vi "dfd_Group Delay_Params Validation.vi"(4 "max pole radius (in)":dbl=0.95 min=0.0, 6 "fs [Hz]":dbl=1.0 format="%.2f", 7 "parameters":T1={"iteration"={"epsilon"=1e-05, "times"=300}, "initial guess"={"iteration times"=5, "seed"=1.0}}, 8 "error in (no error)":errorcluster, 9 "p (in)":i32=128, 10 "dfd_Group Delay_Band Spec":T2[](array[typedef]) {"subband specs"."weight" format="%.2f"}, 11 "order":i32) -> (0 "error out":errorcluster, 1 "p (out)":i32=128, 2 "dfd_Group Delay_Band Spec (dup)":T2[](array[typedef]) {"subband specs"."weight" format="%.2f"}, 3 "max pole radius (out)":dbl)   [LabVIEW 2017, in "NI_DigFilter_Design.lvlib"]
uses:
  <vilib>/addons/Digital Filter Design/NI_DigFilter_Design.lvlib
  <vilib>/addons/Digital Filter Design/_GroupDelay.llb/dfd_Group Delay_Band Spec.ctl
  <vilib>/addons/Digital Filter Design/_Misc.llb/dfd_Error Handlers (Multiple).vi
  <vilib>/addons/Digital Filter Design/NI_DigFilterLicensed.lvlib
panel:
  # "freq"
  # "group delay"
  # "weight"
  # "freq"
  # "group delay"
  # "weight"
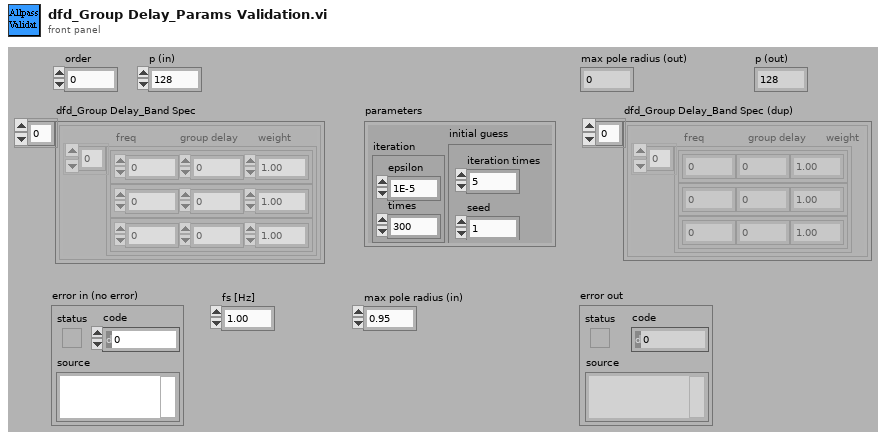
[diagram p1: front panel]
types:
  T1 = cluster{"iteration":cluster{"epsilon":dbl, "times":i32}, "initial guess":cluster{"iteration times":i32, "seed":dbl}}
  T2 = typedef "NI_DigFilterLicensed.lvlib/dfd_Group Delay_Band Spec.ctl" = cluster{"subband specs":cluster{"freq":dbl, "group delay":dbl, "weight":dbl}[]}
  T3 = cluster{"freq":dbl, "group delay":dbl, "weight":dbl}[]
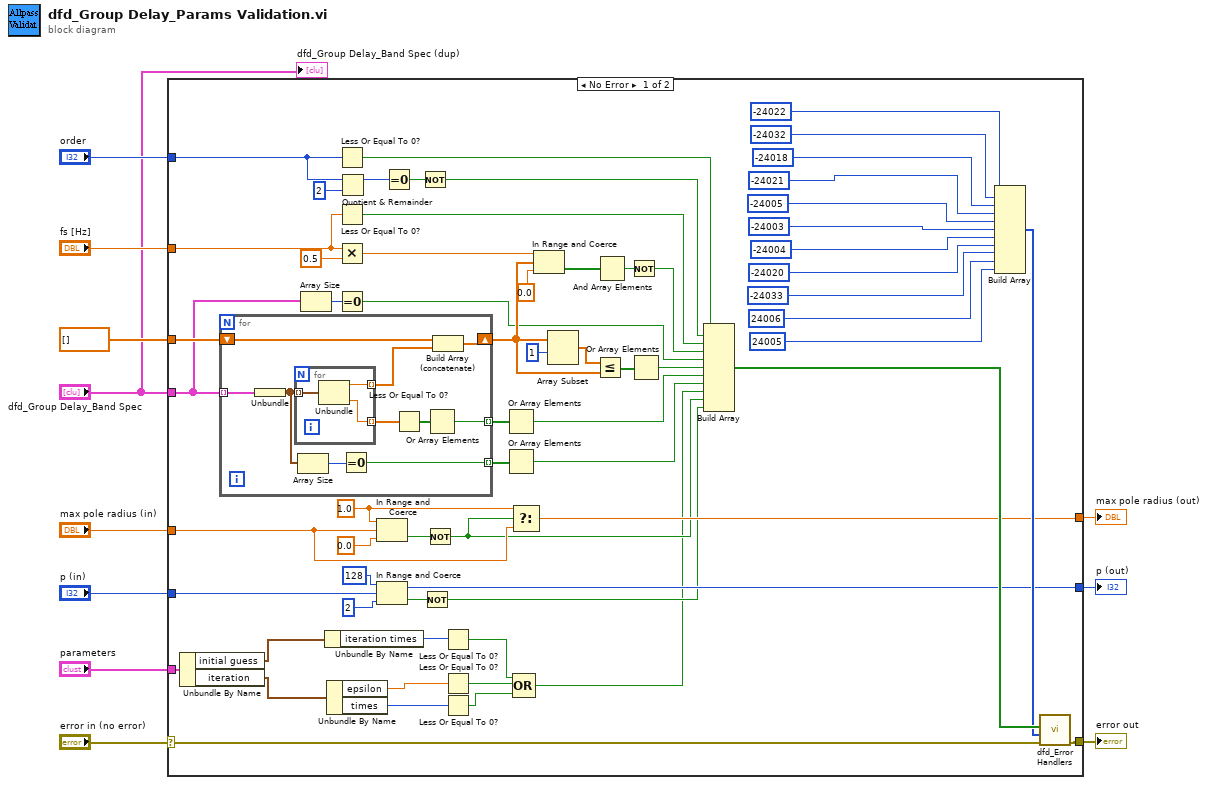
[diagram p0: block diagram]
diagram:
  n1 = case shown="No Error" "error in (no error)" {
    selector: "error in (no error)" -> [w54 w90]
    tunnel: dbl[] [] -> [w75 _]
    tunnel: "fs [Hz]" -> [w62 _]
    tunnel: [w59 w90] -> w9
    tunnel: "p (in)" -> [w44 w91]
    tunnel: [w43 w91] -> w7
    tunnel: "dfd_Group Delay_Band Spec" -> [w42 _]
    tunnel: "order" -> [w28 _]
    tunnel: "max pole radius (in)" -> [w36 w89]
    tunnel: [w34 w89] -> w2
    tunnel: "parameters" -> [w18 _]
    frame No Error {
      w35 = 1.0 ("upper limit")
      n2 = Unbundle By Name(w18) -> ("initial guess"=w20:cluster{"iteration times":i32, "seed":dbl}, "iteration"=w19:cluster{"epsilon":dbl, "times":i32})
      n3 = for {
        tunnel: w42 -> [w85] mode=indexing
        shift-right: [w82] -> w68
        shift-left: w75 -> [w84]
        tunnel: [w79] -> w71 mode=indexing
        tunnel: [w76] -> w48 mode=indexing
        n4 = Unbundle(w85) -> ("subband specs"=w78:T3)
        n5 = for {
          tunnel: w78 -> [w88] mode=indexing
          tunnel: [w87] -> w83 mode=indexing
          tunnel: [w86] -> w81 mode=indexing
          n6 = Unbundle(w88) -> ("freq"=w87:dbl, "weight"=w86:dbl)  [unwired: 1 out]
        }
        n7 = Array Size(array=w78) -> (size(s)=w77:i32)
        n8 = Equal To 0?(x=w77) -> (x = 0?=w76:bool)
        n9 = Less Or Equal To 0?(x=w81) -> (x <= 0?=w80:bool[])
        n10 = Or Array Elements(Boolean array=w80) -> (logical OR=w79:bool)
        n11 = Build Array (concatenate)(w84, w83) -> (w82:dbl[])
      }
      n12 = Array Size(array=w42) -> (size(s)=w41:i32)
      n13 = Unbundle By Name(w20) -> ("iteration times"=w37:i32)
      n14 = Unbundle By Name(w19) -> ("epsilon"=w33:dbl, "times"=w32:i32)
      n15 = Less Or Equal To 0?(x=w28) -> (x <= 0?=w25:bool)
      n16 = Less Or Equal To 0?(x=w62) -> (x <= 0?=w60:bool)
      n17 = Multiply(x=w62, y=0.5) -> (x*y=w64:dbl)
      n18 = Equal To 0?(x=w41) -> (x = 0?=w39:bool)
      n19 = Quotient & Remainder(x=w28, y=2) -> (x-y*floor(x/y)=w26:i32)  [unwired: 1 out]
      n20 = In Range and Coerce(upper limit=w35, x=w36, lower limit=0.0) -> (In Range?=w45:bool)  [unwired: 1 out]
      n21 = In Range and Coerce(upper limit=128, x=w44, lower limit=2) -> (coerced(x)=w43:i32, In Range?=w56:bool)
      n22 = Equal To 0?(x=w26) -> (x = 0?=w24:bool)
      n23 = Not(x=w24) -> (.not. x?=w21:bool)
      n24 = Not(x=w56) -> (.not. x?=w14:bool)
      n25 = Not(x=w45) -> (.not. x?=w13:bool)
      n26 = Less Or Equal To 0?(x=w37) -> (x <= 0?=w31:bool)
      n27 = Less Or Equal To 0?(x=w33) -> (x <= 0?=w30:bool)
      n28 = Less Or Equal To 0?(x=w32) -> (x <= 0?=w29:bool)
      n29 = Or Array Elements(Boolean array=w71) -> (logical OR=w66:bool)
      n30 = Or Array Elements(Boolean array=w48) -> (logical OR=w47:bool)
      n31 = Select(t=w35, s=w13, f=w36) -> (s? t:f=w34:dbl)
      n32 = Compound Arithmetic op=OR(w31, w30, w29) -> (w12:bool)
      n33 = In Range and Coerce(upper limit=w64, x=w68, lower limit=0.0) -> (In Range?=w73:bool[])  [unwired: 1 out]
      n34 = Array Subset(array=w68, index=1) -> (w69:dbl[])  [unwired: 1 in]
      n35 = Less Or Equal?(x=w69, y=w68) -> (x <= y?=w67:bool[])
      n36 = And Array Elements(Boolean array=w73) -> (logical AND=w72:bool)
      n37 = Not(x=w72) -> (.not. x?=w61:bool)
      n38 = Or Array Elements(Boolean array=w67) -> (logical OR=w40:bool)
      n39 = Build Array(w25, w21, w60, w61, w39, w40, w66, w47, w12, w13, w14) -> (w65:bool[])
      n40 = Build Array(-24022 ("ERR_ORDER_LE_ZERO"), -24032 ("ERR_ORDER_ODD"), -24018 ("ERR_FS_LE_ZERO"), -24021 ("ERR_FREQ_RANGE_WRONG"), -24005 ("ERR_EMPTY_BAND"), -24003 ("ERR_BAND_FREQ_SEG_WRONG"), -24004 ("ERR_WEIGHT_LE_ZERO"), -24020 ("ERR_INVALID_BAND"), -24033 ("ERR_INVALID_PARAMETERS"), 24006 ("WRN_RAIUS_RANGE"), 24005 ("WRN_P_RANGE")) -> (w49:i32[])
      n41 = call-poly <vilib>:"dfd_Error Handlers.vi"("error in (no error)"=w54, "error sources"=w49, "condition failed?"=w65) -> ("error out"=w59:errorcluster)  [unwired: 8 out]
    }
    frame Error {
    }
  }
  "error out" <- w9
  "p (out)" <- w7
  "max pole radius (out)" <- w2
  "dfd_Group Delay_Band Spec (dup)" <- "dfd_Group Delay_Band Spec"
